vi "RoomToDbCluster.vi"(8 "error in":errorcluster, 10 "EventTime":timestamp, 11 "Room.lvclass":refnum<class "Room.lvclass">) -> (0 "error out":errorcluster, 2 "RoomEventCluster":T1 {"Flag3" min=0 max=1; "Flag2" min=0 max=1; "Flag1" min=0 max=1; "Flag0" min=0 max=1; "BedVacant" min=0 max=1}, 3 "Room out":refnum<class "Room.lvclass">)   [LabVIEW 2015, in "DatabaseApi.lvlib"]
uses:
  DatabaseApi.lvlib
  LVClasses/Room/Room.lvclass
  TypeDef/Room/RoomTableCluster.ctl
  LVClasses/Room/Room.lvclass/Room.ctl
  LVClasses/Flags/Flags.lvclass/Flags.ctl
  LVClasses/Flags/Flags.lvclass
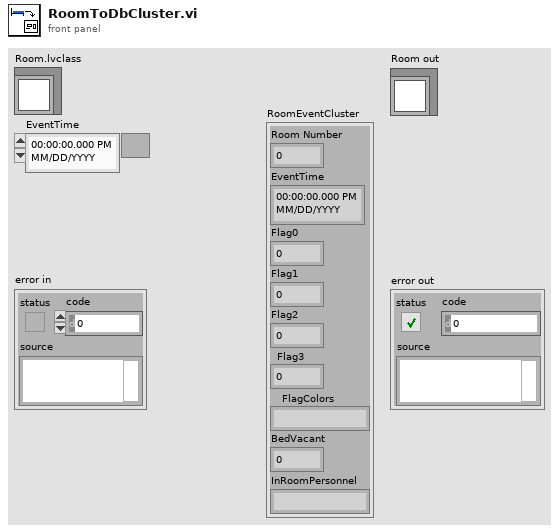
[diagram p1: front panel]
types:
  T1 = typedef "DatabaseApi.lvlib/RoomTableCluster.ctl" = cluster{"Room Number":i32, "EventTime":timestamp, "Flag0":i32, "Flag1":i32, "Flag2":i32, "Flag3":i32, "FlagColors":string, "BedVacant":i32, "InRoomPersonnel":string}
  T2 = typedef "Flags.lvclass/ColorEnum.ctl" = enum8{"Red", "Blue", "Green", "Yellow"}
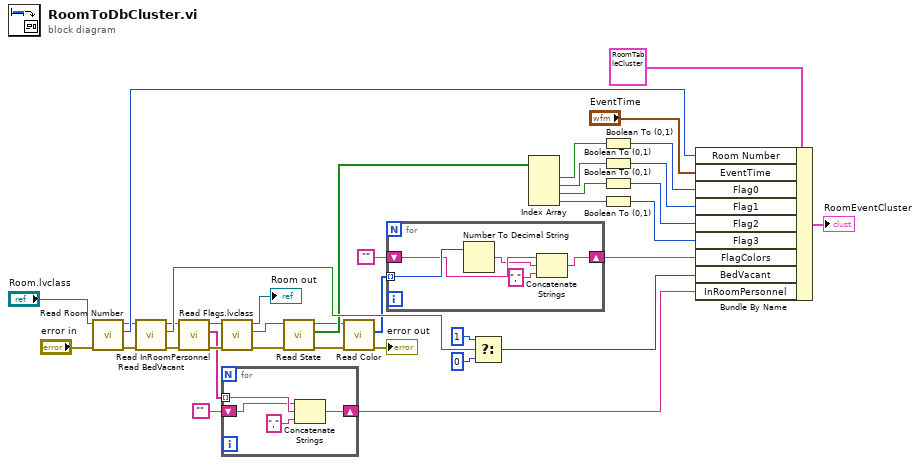
[diagram p0: block diagram]
diagram:
  n1 = call "Read Room Number.vi"("error in (no error)"="error in", "Room in"="Room.lvclass") -> ("error out"=w21:errorcluster, "Room Number"=w34:i32, "Room out"=w22:refnum<class "Room.lvclass">)  [unwired: 7 in]
  n2 = call "Read BedVacant.vi"("error in (no error)"=w21, "Room in"=w22) -> ("error out"=w31:errorcluster, "BedVacant"=w28:bool, "Room out"=w24:refnum<class "Room.lvclass">)  [unwired: 7 in]
  n3 = call "Read InRoomPersonnel.vi"("error in (no error)"=w31, "Room in"=w24) -> ("error out"=w25:errorcluster, "InRoomPersonnel"=w20:string[], "Room out"=w23:refnum<class "Room.lvclass">)  [unwired: 7 in]
  n4 = call "Read Flags.lvclass.vi"("error in (no error)"=w25, "Room in"=w23) -> ("error out"=w27:errorcluster, "Flags.lvclass"=w16:refnum<class "Flags.lvclass">, "Room out"=→"Room out":refnum<class "Room.lvclass">)  [unwired: 7 in]
  n5 = for {
    tunnel: w20 -> [w39] mode=indexing
    shift-right: [w41] -> w18
    shift-left: "" -> [w38]
    n6 = Concatenate Strings(w38, w39, ",") -> (w41:string)
  }
  n7 = call "Read State.vi"("error in (no error)"=w27, "Flags in"=w16) -> ("error out"=w17:errorcluster, "State"=w15:bool[], "Flags out"=w5:refnum<class "Flags.lvclass">)  [unwired: 7 in]
  n8 = call "Read Color.vi"("error in (no error)"=w17, "Flags in"=w5) -> ("error out"=→"error out":errorcluster, "Color"=w2:T2[])  [unwired: 7 in, 1 out]
  n9 = for {
    shift-right: [w46] -> w1
    shift-left: "" -> [w43]
    tunnel: w2 -> [w45] mode=indexing
    n10 = Number To Decimal String(number=w45) -> (decimal integer string=w42:string)  [unwired: 1 in]
    n11 = Concatenate Strings(w43, w42, ",") -> (w46:string)
  }
  n12 = Select(t=1 ("BedVacant"), s=w28, f=0 ("BedVacant")) -> (s? t:f=w4:i32)
  n13 = Index Array(array=w15) -> (element #1=w14:bool, element #2=w11:bool, element #3=w10:bool, element #4=w8:bool)  [unwired: 4 in]
  n14 = Boolean To (0,1)(Boolean=w14) -> (0, 1=w13:i16)
  n15 = Boolean To (0,1)(Boolean=w11) -> (0, 1=w12:i16)
  n16 = Boolean To (0,1)(Boolean=w10) -> (0, 1=w9:i16)
  n17 = Boolean To (0,1)(Boolean=w8) -> (0, 1=w7:i16)
  n18 = Bundle By Name(cluster=T1 {"Room Number"=0, "EventTime"=timestamp(0 s since 1904-01-01), "Flag0"=0, "Flag1"=0, "Flag2"=0, "Flag3"=0, "FlagColors"="", "BedVacant"=0, "InRoomPersonnel"=""} ("Cluster"), "Room Number"=w34, "EventTime"="EventTime", "Flag0"=w13, "Flag1"=w12, "Flag2"=w9, "Flag3"=w7, "FlagColors"=w1, "BedVacant"=w4, "InRoomPersonnel"=w18) -> (→"RoomEventCluster":T1)
